vi "New QuVI.vi"   [LabVIEW 2016]
panel:
  # "QuVI Template\n\nOpen the block diagram (Ctrl+E) and start circuit composing"
types:
  T1 = typedef "Circuit Cluster.ctl" = cluster{"Loop No":i32, "Wire":cluster{"No":i32, "Depth":i32, "Hold":i32[][], "Permits":refnum<notifier>}, "Size":refnum<queue>, "Composition":refnum<queue>, "Gate class":refnum<class "GateAbst.lvclass">}
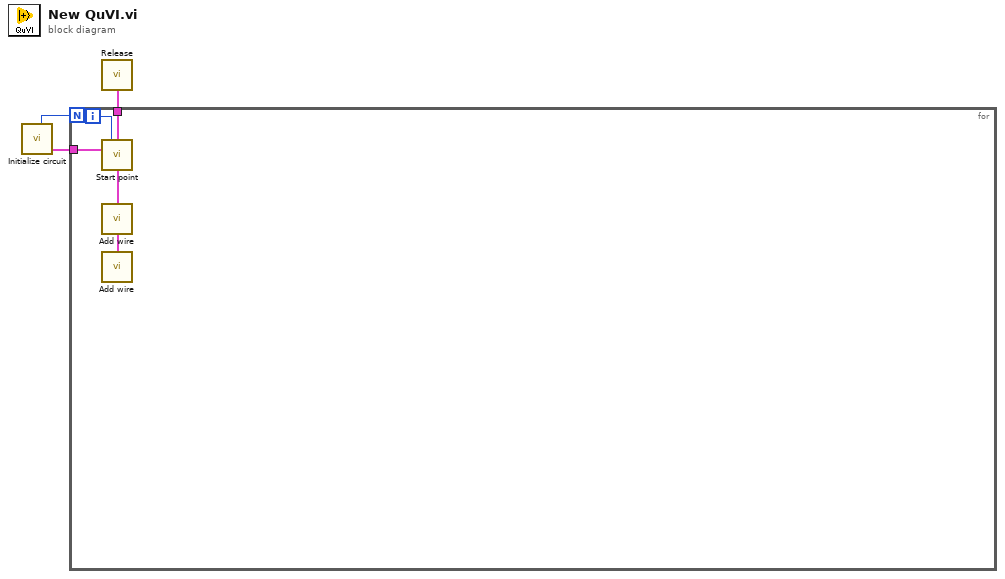
[diagram p0: block diagram]
diagram:
  n1 = call "Initialize circuit.vi"() -> ("N"=w3:i32, "Circuit cluster"=w2:T1)  [unwired: 8 in]
  n2 = for {
    N: w3 -> [_]
    tunnel: w2 -> [w8]
    tunnel: [w5] -> w1
    i -> [w4]
    n3 = call "Start point.vi"("Loop No"=w4, "Circuit cluster in"=w8) -> ("Up circuit cluster out"=w5:T1, "Down circuit cluster out"=w7:T1)  [unwired: 12 in]
    n4 = call "Add wire.vi"("Circuit cluster in"=w7) -> ("Circuit cluster out"=w6:T1)  [unwired: 13 in, 1 out]
    n5 = call "Add wire.vi"("Circuit cluster in"=w6) -> ()  [unwired: 13 in, 2 out]
  }
  n6 = call "Release.vi"("Circuit cluster in"=w1) -> ()  [unwired: 15 in]
